vi "Read_valve_Pos_fr_server.vi"() -> (0 "Valve Error Info":string, 1 "Output Value":dbl format="%.2f")   [LabVIEW 2014]
panel:
  out "Repeat Number":i32
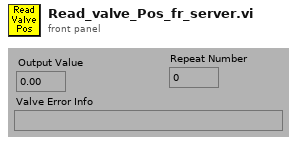
[diagram p1: front panel]
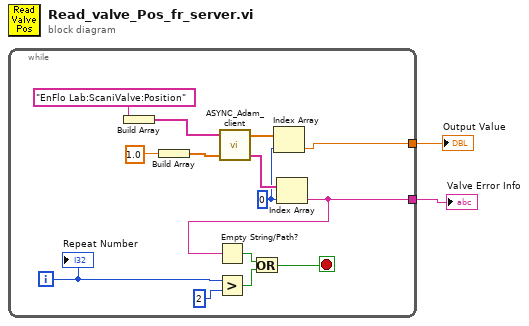
[diagram p0: block diagram]
diagram:
  n1 = while {
    tunnel: [w9] -> w2
    tunnel: [w8] -> w1
    i -> [w7]
    stop <- w3 stop-if-true
    w10 = 0 ("Index")
    n2 = Build Array("EnFlo Lab:ScaniValve:Position") -> (w15:string[])
    n3 = Build Array(1.0) -> (w13:dbl[])
    n4 = Greater?(x=w7, y=2) -> (0:w5:bool)
    n5 = call "ASYNC_Adam_client.vi"("Values"=w13, "Channel Names"=w15) -> ("Scan Comments"=w11:string[], "Calibrated Units"=w12:dbl[])  [unwired: 1 in]
    n6 = Index Array(array=w12, index=w10) -> (element=w9:dbl)
    n7 = Index Array(array=w11, index=w10) -> (element=w8:string)
    n8 = Empty String/Path?(string/path=w8) -> (empty?=w4:bool)
    n9 = Or(x=w4, y=w5) -> (x .or. y?=w3:bool)
    "Repeat Number" <- w7
  }
  "Output Value" <- w2
  "Valve Error Info" <- w1
